vi "Category Manager.vi"() -> ()   [LabVIEW 2018]
panel:
  out "Array":i32[](array[numeric])
  in  "Delete":bool
  in  "OK":bool
  in  "Add":bool
  in  "Category Name":string
  in  "Category Table":string[][](table)
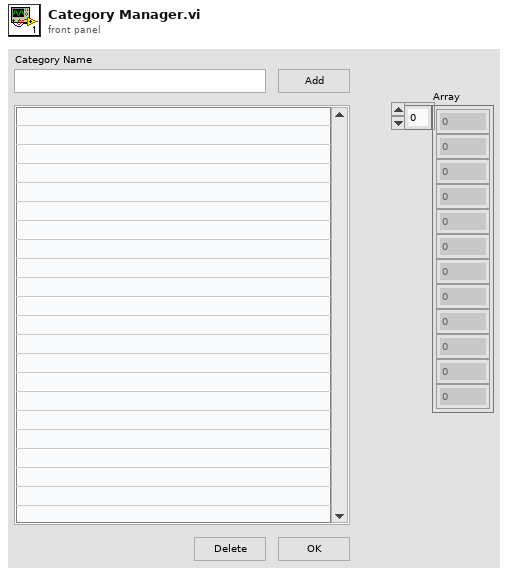
[diagram p1: front panel]
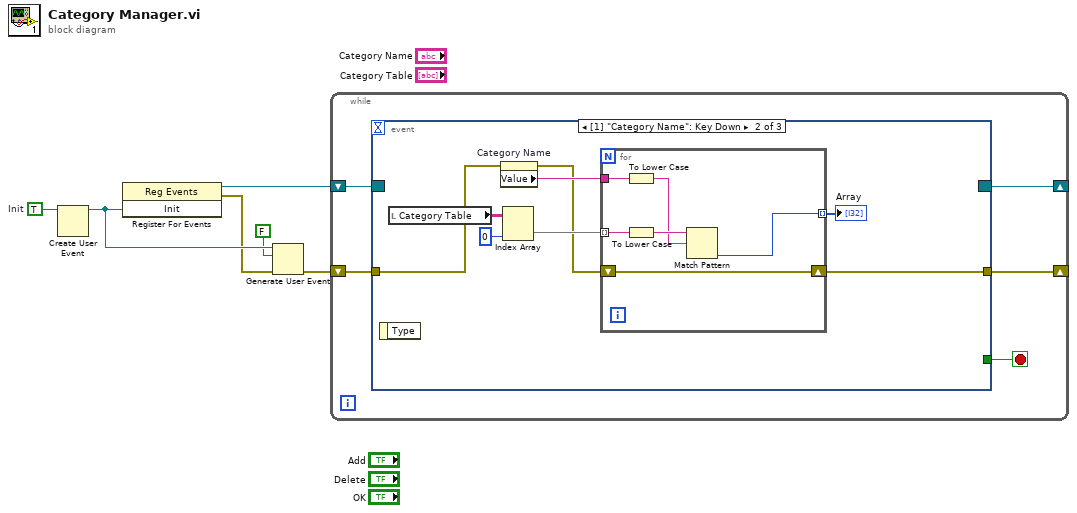
[diagram p0: block diagram]
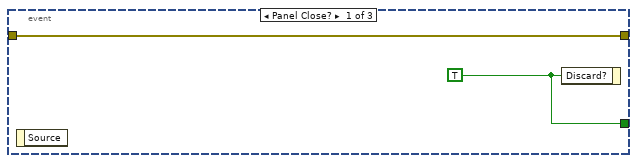
[diagram p2: hidden frame]
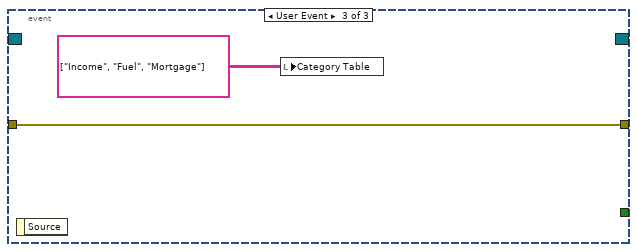
[diagram p3: hidden frame]
diagram:
  w6 = TRUE  # Init
  n1 = Create User Event(user event datatype=w6) -> (user event=w4:refnum<user-event>)  [unwired: 1 in, 1 out]
  n2 = register-events(w4) -> (reference out=w5:refnum<event-registration>, error out=w3:errorcluster)  [unwired: 2 in]
  n3 = Generate User Event(user event=w4, event data cluster=FALSE ("event data"), error in=w3) -> (error out=w2:errorcluster)  [unwired: 1 in, 1 out]
  n4 = while {
    shift-right: [w7] -> _
    shift-left: w5 -> [w10]
    shift-right: [w8] -> _
    shift-left: w2 -> [w9]
    stop <- w11 stop-if-true
    n5 = event shown="[1] \"Category Name\": Key Down" {
      selector: w10 -> [_ _ _]
      dyn-events: [_ _ _] -> w7
      timeout: _ -> [_ _ _]
      tunnel: [w13 _ _] -> w11
      tunnel: w9 -> [w12 w14 w28]
      tunnel: [w12 w19 w28] -> w8
      event Panel Close? {
        w13 = TRUE ("Discard?")
        n6 = event-data() -> ()  [unwired: 1 in, 1 out]
        n7 = event-data("Discard?"=w13) -> ()  [unwired: 1 in, 1 out]
      }
      event "Category Name": Key Down {
        n8 = event-data() -> ()  [unwired: 1 in, 1 out]
        n9 = local read "Category Table"() -> (w21:string[][])
        n10 = property on="Category Name" class="Str"(error in=w14) -> (error out=w15:errorcluster, "Value"=w16:string)  [unwired: 1 in, 1 out]
        n11 = Index Array(array=w21, index (col)=0 ("disabled index (col)")) -> (element=w18:string[])  [unwired: 1 in]
        n12 = for {
          shift-right: [w22] -> w19
          shift-left: w15 -> [w22]
          tunnel: w18 -> [w27] mode=indexing
          tunnel: w16 -> [w26]
          tunnel: [w23] -> w17 mode=indexing
          n13 = To Lower Case(string=w26) -> (all lower case string=w24:string)
          n14 = To Lower Case(string=w27) -> (all lower case string=w25:string)
          n15 = Match Pattern(string=w25, regular expression=w24) -> (offset past match=w23:i32)  [unwired: 1 in, 3 out]
        }
        "Array" <- w17
      }
      event User Event {
        n16 = event-data() -> ()  [unwired: 1 in, 1 out]
        n17 = local write "Category Table"(string[][] [["Income"], ["Fuel"], ["Mortgage"]] ("Category Table")) -> ()
      }
    }
  }
